vi "TWM Client Cmd Get Status.vi"(5 "timeout [ms] (3000)":i32=3000, 7 "end of packet key":string="TWM:command:EndOfPacket", 8 "error in":errorcluster, 11 "handle":i32) -> (0 "error out":errorcluster, 1 "error message":string, 2 "ready?":bool, 3 "handle out":i32, 4 "status string":string)   [LabVIEW 2020, in "TWM Client.lvlib"]
doc: "Write Get status command packet to TWM server. Get answer. Returns 'Ready?', when server is ready to do stuff. Also returns optional error text message from server. It will generate error if error message was not empty."
uses:
  TWM Client.lvlib
  GetString.vi
  Get 1D String.vi
  <vilib>/Utility/error.llb/Error Cluster From Error Code.vi
  <vilib>/ErrorRing/Error Ring.xnode
  infolib.lvlib
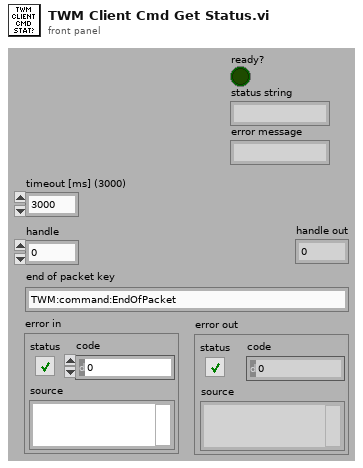
[diagram p1: front panel]
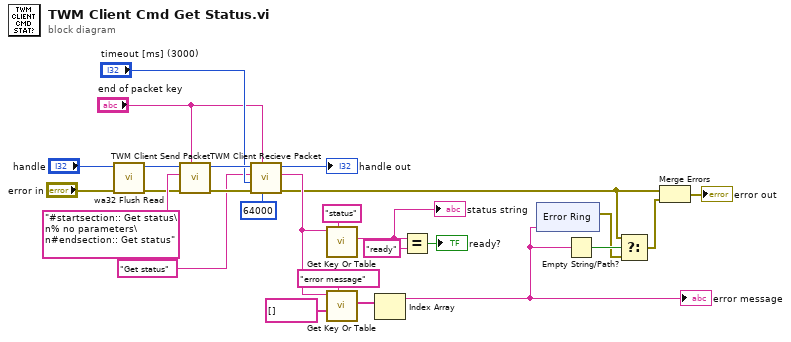
[diagram p0: block diagram]
diagram:
  n1 = call "wa32 Flush Read.vi"("error in"="error in", "handle"="handle") -> ("error out"=w3:errorcluster, "handle out"=w2:i32)  [unwired: 7 in, 1 out]
  n2 = call "TWM Client Send Packet.vi"("end of packet key"="end of packet key", "error in"=w3, "command string"="#startsection:: Get status\n% no parameters\n#endsection:: Get status", "handle"=w2) -> ("error out"=w19:errorcluster, "handle out"=w17:i32)  [unwired: 6 in]
  n3 = call "TWM Client Recieve Packet.vi"("max message length (1024)"=64000, "end of packet key"="end of packet key", "error in"=w19, "timeout [ms] (5000 ms)"="timeout [ms] (3000)", "message header (empty)"="Get status" ("key string"), "handle in"=w17) -> ("error out"=w7:errorcluster, "message data"=w12:string, "handle out"=→"handle out":i32)  [unwired: 3 in]
  n4 = call-poly "Get Key Or Table.vi"("key description"="status", "info data"=w12) -> ("value"=w24:string)  [unwired: 6 in, 3 out]
  "status string" <- w24
  n5 = call-poly "Get Key Or Table.vi"("key description"="error message", "string"=string[] [], "info data"=w12) -> ("value"=w20:string[])  [unwired: 5 in, 3 out]
  n6 = Index Array(array=w20) -> (element=w9:string)  [unwired: 1 in]
  "error message" <- w9
  n7 = Equal?(x=w24, y="ready") -> (x = y?=→"ready?":bool)
  n8 = xnode "Error Ring"("parameter 0"=w9) -> ("error out"=w8:errorcluster)
  n9 = Empty String/Path?(string/path=w9) -> (empty?=w10:bool)
  n10 = Select(t=w7, s=w10, f=w8) -> (s? t:f=w6:errorcluster)
  n11 = Merge Errors(w7, w6) -> (→"error out":errorcluster)
